vi "MecaWheelPos_Sub.vi"(9 "In MECA_WHEEL_POSITIONS 2":T1 {"RearRight" format="%19.3f"; "RearLeft" format="%19.3f"; "FrontRight" format="%19.3f"; "FrontLeft" format="%19.3f"}, 11 "In MECA_WHEEL_POSITIONS 1":T1 {"RearRight" format="%19.3f"; "RearLeft" format="%19.3f"; "FrontRight" format="%19.3f"; "FrontLeft" format="%19.3f"}) -> (3 "MECA_WHEEL_POSITIONS":T1 {"RearRight" format="%19.3f"; "RearLeft" format="%19.3f"; "FrontRight" format="%19.3f"; "FrontLeft" format="%19.3f"})   [LabVIEW 2019, in "Trajectory_Library.lvlib"]
doc: "Subtract two MecanumDriveWheelPosition data structures to create a delta MecanumDriveWheelPosition\n\nReturns MecaWheelPos1 - MecaWheelPos2\n\nParameters:\n - in Meca_wheel_Position1- Data structure\n - in Meca_wheel_Position2- Data structure\n\nReturns:\n - Meca_wheel_Position- Data structure"
uses:
  Trajectory_Library.lvlib
  TypeDef/MECA_WHEEL_POSITIONS.ctl
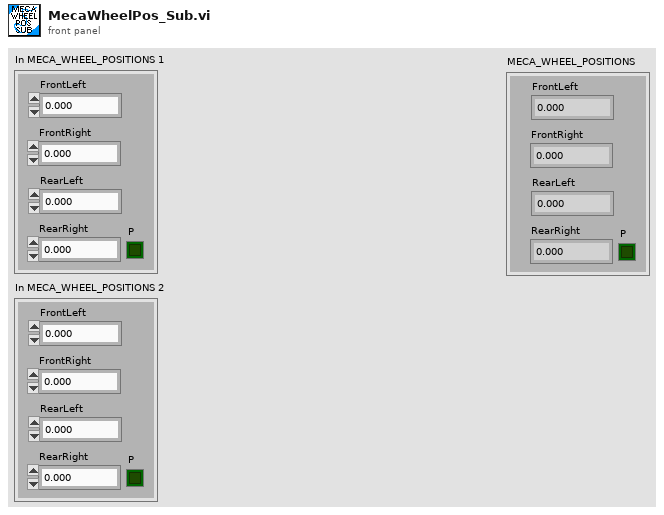
[diagram p1: front panel]
types:
  T1 = typedef "Trajectory_Library.lvlib/MECA_WHEEL_POSITIONS.ctl" = cluster{"FrontLeft":dbl, "FrontRight":dbl, "RearLeft":dbl, "RearRight":dbl, "P":bool}
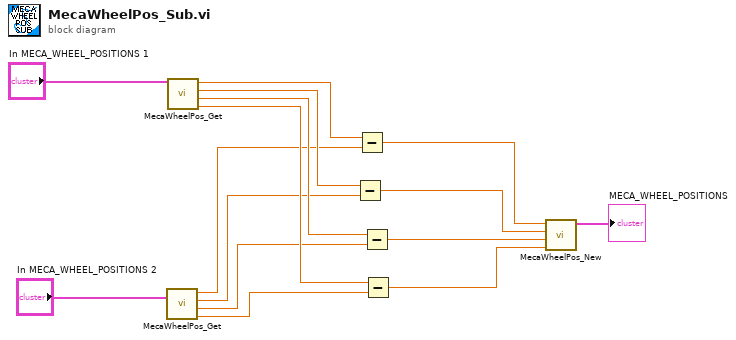
[diagram p0: block diagram]
diagram:
  n1 = call "MecaWheelPos_Get.vi"("MECA_WHEEL_POSITIONS"="In MECA_WHEEL_POSITIONS 2") -> ("RearRightPosition"=w1:dbl, "RearLeftPosition"=w2:dbl, "FrontRightPosition"=w3:dbl, "FrontLeftPosition"=w4:dbl)  [unwired: 7 in]
  n2 = call "MecaWheelPos_Get.vi"("MECA_WHEEL_POSITIONS"="In MECA_WHEEL_POSITIONS 1") -> ("RearRightPosition"=w5:dbl, "RearLeftPosition"=w6:dbl, "FrontRightPosition"=w7:dbl, "FrontLeftPosition"=w8:dbl)  [unwired: 7 in]
  n3 = Subtract(x=w7, y=w3) -> (x-y=w11:dbl)
  n4 = Subtract(x=w8, y=w4) -> (x-y=w12:dbl)
  n5 = Subtract(x=w6, y=w2) -> (x-y=w10:dbl)
  n6 = Subtract(x=w5, y=w1) -> (x-y=w9:dbl)
  n7 = call "MecaWheelPos_New.vi"("RearRightPosition"=w9, "RearLeftPosition"=w10, "FrontRightPosition"=w11, "FrontLeftPosition"=w12) -> ("MECA_WHEEL_POSITIONS"=→"MECA_WHEEL_POSITIONS":T1)  [unwired: 7 in]
